vi "svfa_Linear OneShot or AutoRestart Averaging Done.vi"(6 "averaging parameters":T2={"averaging mode"=enum."No averaging", "weighting mode"=enum."Linear", "number of averages"=10, "linear mode"=enum."Auto restart"}, 7 "averaging done":bool, 8 "error in (no error)":errorcluster) -> (0 "error out":errorcluster, 4 "processing control":T1(ring))   [LabVIEW 2017]
doc: "This VI sets the restart averaging and retrieve previous spectrum flags according to the linear weighting mode."
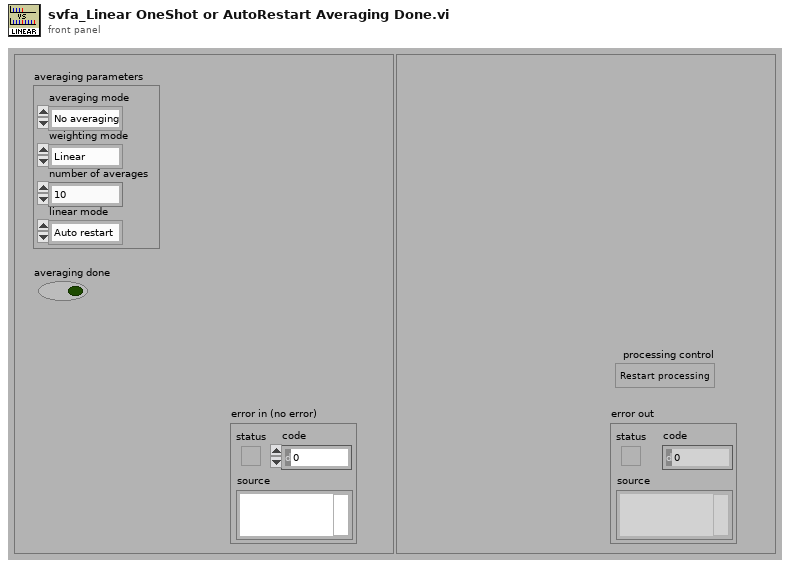
[diagram p1: front panel]
types:
  T1 = enum16{"Restart processing", "Continue processing", "Skip processing"}
  T2 = cluster{"averaging mode":enum16{"No averaging", "Vector averaging", "RMS averaging", "Peak hold"}, "weighting mode":enum16{"Linear", "Exponential"}, "number of averages":u32, "linear mode":enum16{"One shot", "Auto restart"}}
  T3 = enum16{"No averaging", "Vector averaging", "RMS averaging", "Peak hold"}
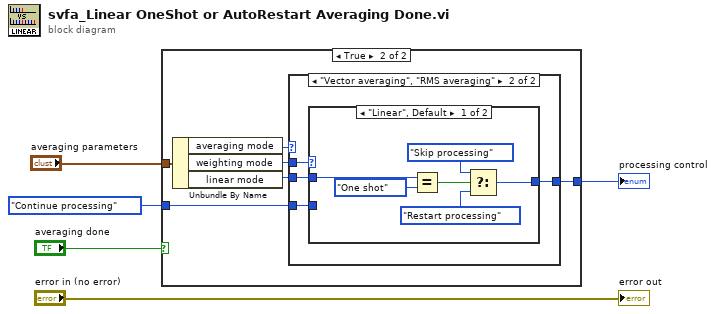
[diagram p0: block diagram]
diagram:
  n1 = case shown="True" "averaging done" {
    tunnel: "averaging parameters" -> [_ w11]
    tunnel: [w6 w10] -> w2
    tunnel: T1."Continue processing" ("processing control") -> [w6 w7]
    frame False {
    }
    frame True {
      n2 = Unbundle By Name(w11) -> ("averaging mode"=w12:T3, "weighting mode"=w9:enum16{"Linear", "Exponential"}, "linear mode"=w8:enum16{"One shot", "Auto restart"})
      n3 = case shown="\"Vector averaging\", \"RMS averaging\"" w12 {
        tunnel: [w13 w17] -> w10
        tunnel: w9 -> [_ w16]
        tunnel: w8 -> [_ w15]
        tunnel: w7 -> [w13 w14]
        frame "No averaging", "Peak hold", Default {
        }
        frame "Vector averaging", "RMS averaging" {
          n4 = case shown="\"Linear\", Default" w16 {
            tunnel: [w19 w24] -> w17
            tunnel: w15 -> [w18 _]
            tunnel: w14 -> [_ w24]
            frame "Linear", Default {
              n5 = Equal?(x=w18, y=enum16{"One shot", "Auto restart"}."One shot") -> (x = y?=w22:bool)
              n6 = Select(t=T1."Skip processing" ("processing control"), s=w22, f=T1."Restart processing" ("processing control")) -> (s? t:f=w19:T1)
            }
            frame "Exponential" {
            }
          }
        }
      }
    }
  }
  "processing control" <- w2
  "error out" <- "error in (no error)"
